vi "CubicHermiteSpline_makeHermiteBasis.vi"() -> (3 "HermiteBasis":T1)   [LabVIEW 2019, in "Trajectory_Library.lvlib"]
doc: "Returns the hermite basis matrix for cubic hermite spline interpolation.\n\nParameters:\n - none -\n\nReturns:\n - HermiteBasis - The hermite basis matrix for cubic hermite spline interpolation."
uses:
  Trajectory_Library.lvlib
  <vilib>/Analysis/Matrix/Datatypes/RealMatrix.ctl
  <vilib>/Analysis/Matrix/NI_Matrix.lvlib
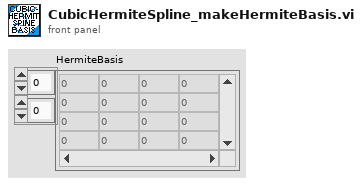
[diagram p1: front panel]
types:
  T1 = typedef "NI_Matrix.lvlib/RealMatrix.ctl" = dbl[][]
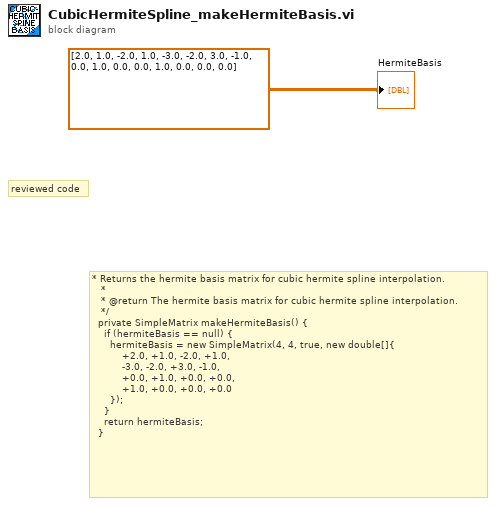
[diagram p0: block diagram]
diagram:
  # "reviewed code"
  # "* Returns the hermite basis matrix for cubic hermite spline interpolation.\n   *\n   * @return The hermite basis matrix for cubic hermite spline interpolation.\n   */\n  private SimpleMatrix makeHermiteBasis() {\n    if (hermiteBasis == null) {\n      hermiteBasis = new SimpleMatrix(4, 4, true, new double[]{\n          +2.0, +1.0, -2.0, +1.0,\n          -3.0, -2.0, +3.0, -1.0,\n          +0.0, +1.0, +0.0, +0.0,\n          +1.0, +0.0, +0.0, +0.0\n      });\n    }\n    return hermiteBasis;\n  }"
  "HermiteBasis" <- T1 [[2.0, 1.0, -2.0, 1.0], [-3.0, -2.0, 3.0, -1.0], [0.0, 1.0, 0.0, 0.0], [1.0, 0.0, 0.0, 0.0]] ("HermiteBasis")
